vi "PolyRemSlope.vi"(11 "PolysIn":T1[](array[typedef])) -> (3 "PolysOut":cluster{cluster{"X":sgl, "Y":sgl}[]}[](array[cluster]))   [LabVIEW 2014]
uses:
  TypeDefs/Poly2DwSlope.ctl
  TypeDefs/Point2DwSlope.ctl
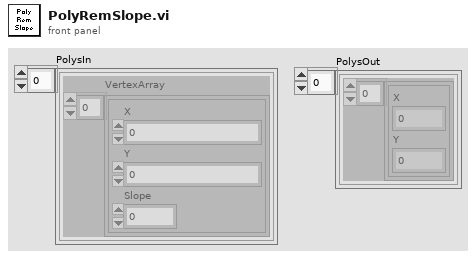
[diagram p1: front panel]
types:
  T1 = typedef "Poly2DwSlope.ctl" = cluster{"VertexArray":T2[]}
  T2 = typedef "Point2DwSlope.ctl" = cluster{"X":sgl, "Y":sgl, "Slope":dbl}
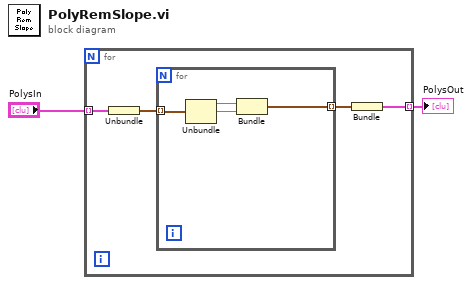
[diagram p0: block diagram]
diagram:
  n1 = for {
    tunnel: "PolysIn" -> [w6] mode=indexing
    tunnel: [w3] -> w1 mode=indexing
    n2 = Unbundle(w6) -> ("VertexArray"=w5:T2[])
    n3 = for {
      tunnel: w5 -> [w10] mode=indexing
      tunnel: [w7] -> w4 mode=indexing
      n4 = Unbundle(w10) -> ("X"=w9:sgl, "Y"=w8:sgl)  [unwired: 1 out]
      n5 = Bundle("X"=w9, "Y"=w8) -> (w7:cluster{"X":sgl, "Y":sgl})  [unwired: 1 in]
    }
    n6 = Bundle(w4) -> (w3:cluster{cluster{"X":sgl, "Y":sgl}[]})  [unwired: 1 in]
  }
  "PolysOut" <- w1
